vi "dashboard_to_send.vi"(1 "In":T1) -> (0 "Output":u8[](array[numeric]))   [LabVIEW 2022 SP3]
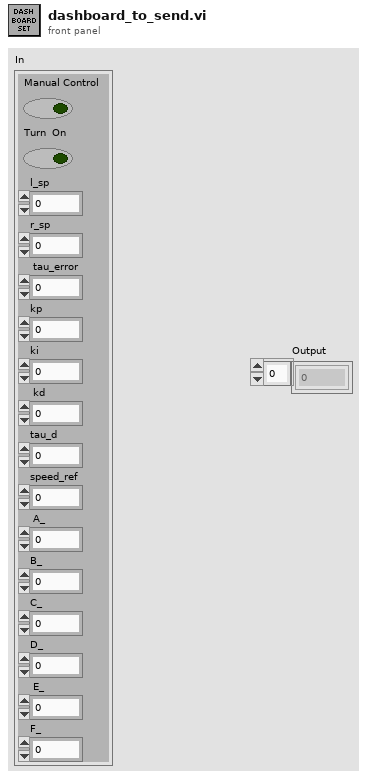
[diagram p1: front panel]
types:
  T1 = cluster{"Manual Control":bool, "Turn  On":bool, "l_sp":dbl, "r_sp":dbl, " tau_error":dbl, "kp":dbl, "ki":dbl, " kd":dbl, "tau_d":dbl, "speed_ref":dbl, " A_":dbl, "B_":dbl, "C_":dbl, "D_":dbl, " E_":dbl, "F_":dbl}
  T2 = cluster{u8, u8, i16, i16, u16, u16, u16, u16, u16, u16, i16, i16, i16, i16, i16, i16}
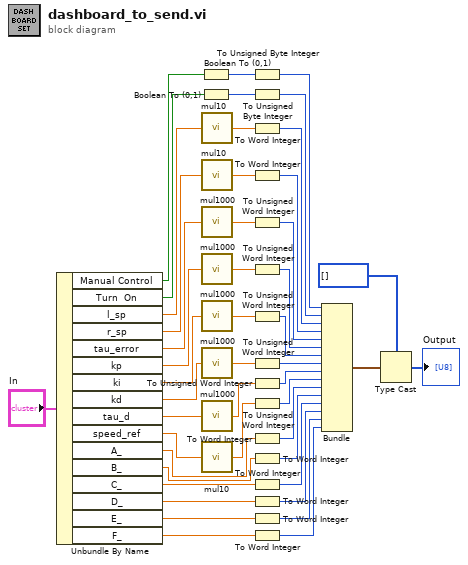
[diagram p0: block diagram]
diagram:
  n1 = Unbundle By Name("In") -> ("Manual Control"=w16:bool, "Turn  On"=w15:bool, "l_sp"=w14:dbl, "r_sp"=w13:dbl, "tau_error"=w12:dbl, "kp"=w11:dbl, "ki"=w10:dbl, "kd"=w9:dbl, "tau_d"=w8:dbl, "speed_ref"=w7:dbl, "A_"=w6:dbl, "B_"=w5:dbl, "C_"=w4:dbl, "D_"=w3:dbl, "E_"=w2:dbl, "F_"=w1:dbl)
  n2 = Boolean To (0,1)(Boolean=w16) -> (0, 1=w35:i16)
  n3 = Boolean To (0,1)(Boolean=w15) -> (0, 1=w34:i16)
  n4 = call "mul10.vi"("x"=w14) -> ("y"=w33:dbl)
  n5 = call "mul10.vi"("x"=w13) -> ("y"=w32:dbl)
  n6 = call "mul1000.vi"("x"=w12) -> ("y"=w29:dbl)
  n7 = call "mul1000.vi"("x"=w11) -> ("y"=w19:dbl)
  n8 = call "mul1000.vi"("x"=w10) -> ("y"=w22:dbl)
  n9 = call "mul1000.vi"("x"=w9) -> ("y"=w21:dbl)
  n10 = call "mul1000.vi"("x"=w8) -> ("y"=w20:dbl)
  n11 = call "mul10.vi"("x"=w7) -> ("y"=w18:dbl)
  n12 = To Unsigned Byte Integer(number=w35) -> (unsigned 8bit integer=w45:u8)
  n13 = To Unsigned Byte Integer(number=w34) -> (unsigned 8bit integer=w44:u8)
  n14 = To Word Integer(number=w33) -> (16bit integer=w43:i16)
  n15 = To Word Integer(number=w32) -> (16bit integer=w42:i16)
  n16 = To Unsigned Word Integer(number=w29) -> (unsigned 16bit integer=w28:u16)
  n17 = To Unsigned Word Integer(number=w19) -> (unsigned 16bit integer=w27:u16)
  n18 = To Unsigned Word Integer(number=w22) -> (unsigned 16bit integer=w26:u16)
  n19 = To Unsigned Word Integer(number=w21) -> (unsigned 16bit integer=w25:u16)
  n20 = To Unsigned Word Integer(number=w20) -> (unsigned 16bit integer=w24:u16)
  n21 = To Unsigned Word Integer(number=w18) -> (unsigned 16bit integer=w23:u16)
  n22 = To Word Integer(number=w6) -> (16bit integer=w41:i16)
  n23 = To Word Integer(number=w5) -> (16bit integer=w40:i16)
  n24 = To Word Integer(number=w4) -> (16bit integer=w39:i16)
  n25 = To Word Integer(number=w3) -> (16bit integer=w38:i16)
  n26 = To Word Integer(number=w2) -> (16bit integer=w37:i16)
  n27 = To Word Integer(number=w1) -> (16bit integer=w36:i16)
  n28 = Bundle(w45, w44, w43, w42, w28, w27, w26, w25, w24, w23, w41, w40, w39, w38, w37, w36) -> (w30:T2)  [unwired: 1 in]
  n29 = Type Cast(type=u8[] [], x=w30) -> (*(type *) &x=→"Output":u8[])
